vi "BuildRelease_RecompileOpenGDS.vi"() -> ()   [LabVIEW 2020]
uses:
  <vilib>/Utility/config.llb/Read Key (String).vi
  <vilib>/Utility/config.llb/NI_LVConfig.lvlib
panel:
  out "error IO":errorcluster
  out "File":path
  out "Opening":i32
  out "Saving Libraries":i32
  out "Saving Classes":i32
  out "Saving VIs":i32
  out "resulting string":string
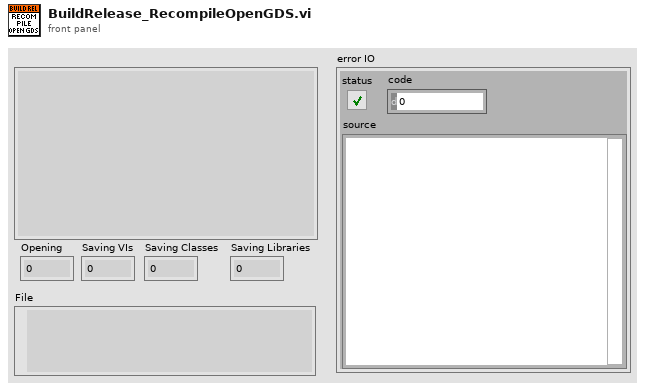
[diagram p1: front panel]
types:
  T1 = cluster{"PID":string, "SpecPath":path, "Files":string[], "BuildPath":path, "InstallerPath":path, "Start":timestamp, "LogFile":path, "AllVIs":refnum<vi>[], "Locked":string[], "Modified":string[], "Bad":string[], "SaveAllError":string[]}
  T2 = enum32{"Bad", "Idle", "Run top level", "Running"}
  T3 = typedef "NI_LVConfig.lvlib/Config Data RefNum.ctl" = refnum<k1>
  T4 = enum32{"invalid lock state", "Not Locked", "Locked (No Password)", "Password-protected"}
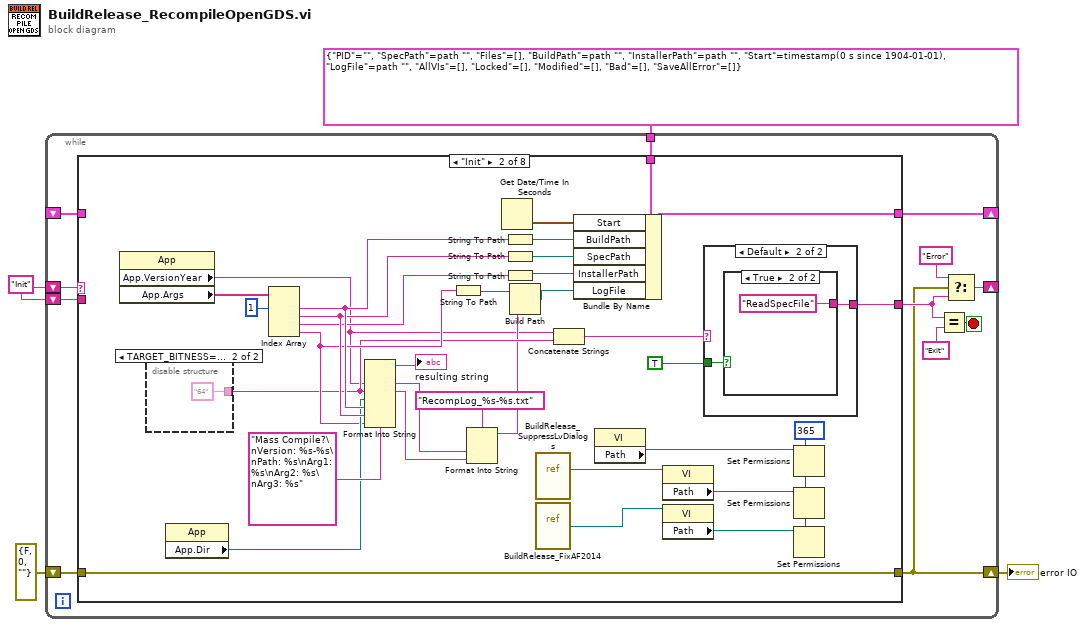
[diagram p0: block diagram]
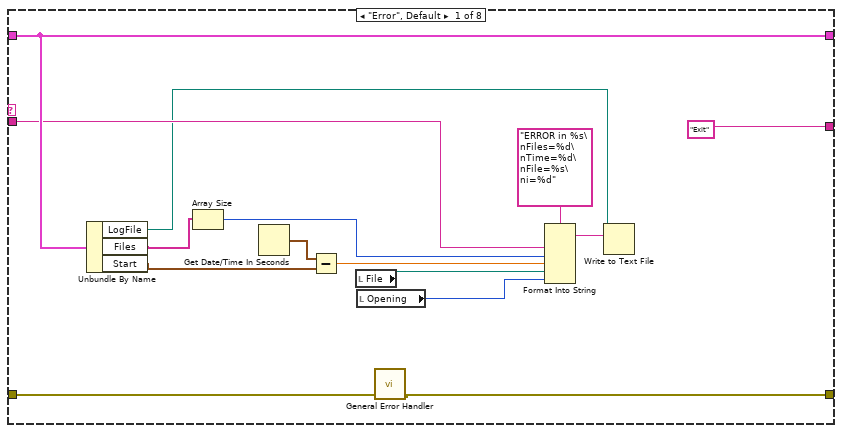
[diagram p2: hidden frame]
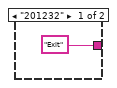
[diagram p3: hidden frame]
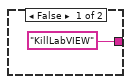
[diagram p4: hidden frame]
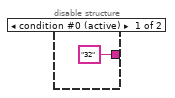
[diagram p5: hidden frame]
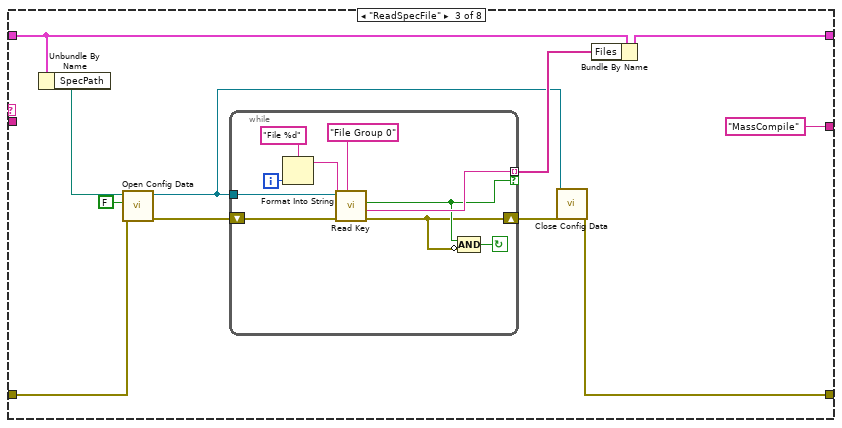
[diagram p6: hidden frame]
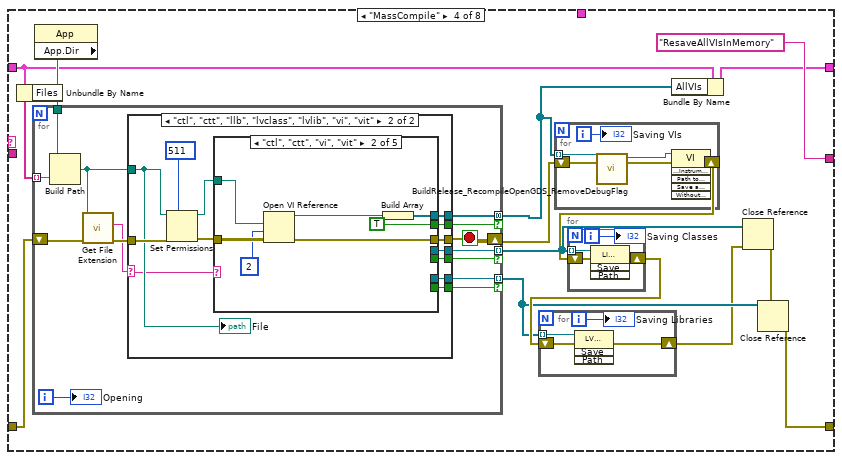
[diagram p7: hidden frame]
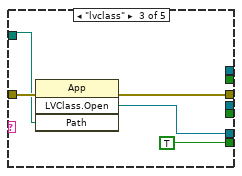
[diagram p10: hidden frame]
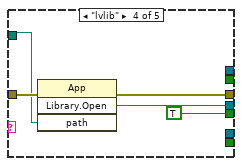
[diagram p11: hidden frame]
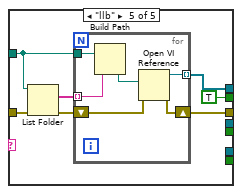
[diagram p12: hidden frame]
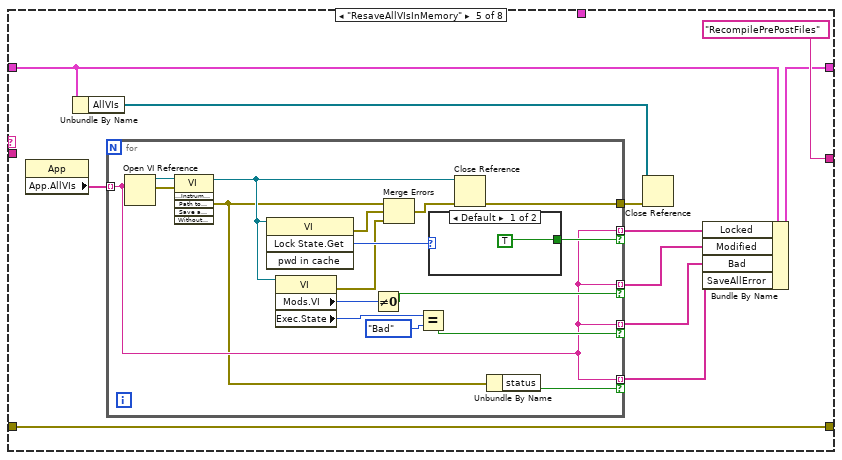
[diagram p13: hidden frame]
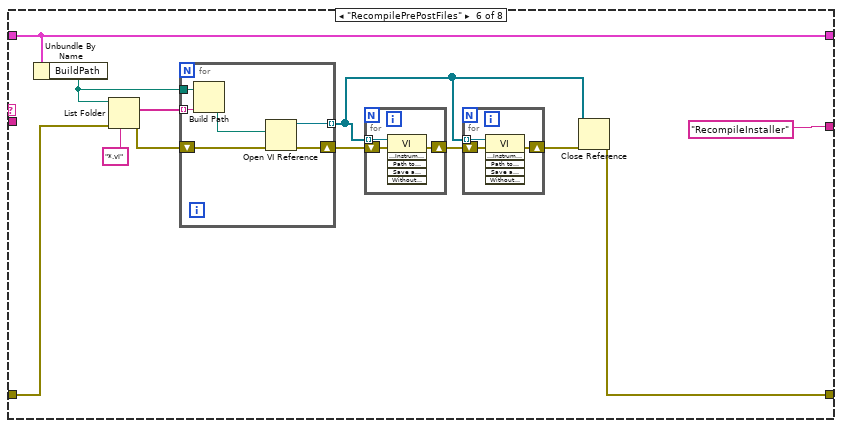
[diagram p15: hidden frame]
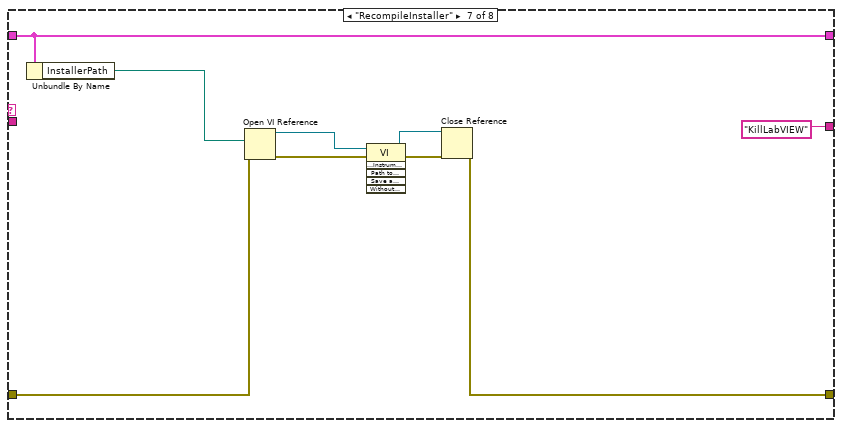
[diagram p16: hidden frame]
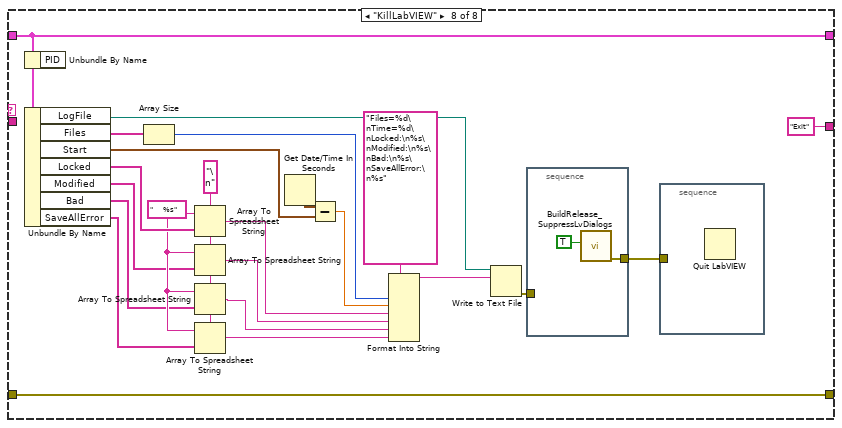
[diagram p17: hidden frame]
diagram:
  w2 = "Init"
  n1 = while {
    shift-right: [w9] -> w1
    shift-left: errorcluster {"status"=FALSE, "code"=0, "source"=""} ("error IO") -> [w16]
    shift-right: [w14] -> _
    shift-left: w2 -> [w15]
    shift-right: [w8] -> _
    shift-left: _ -> [w7]
    tunnel: T1 {"PID"="", "SpecPath"=path "", "Files"=[], "BuildPath"=path "", "InstallerPath"=path "", "Start"=timestamp(0 s since 1904-01-01), "LogFile"=path "", "AllVIs"=[], "Locked"=[], "Modified"=[], "Bad"=[], "SaveAllError"=[]} -> [w6]
    shift-left: w2 -> [w5]
    stop <- w13 stop-if-true
    n2 = case shown="\"Init\"" w15 {
      tunnel: w16 -> [w30 w61 w73 w99 w183 w213 w235 w262]
      tunnel: [w17 w61 w71 w98 w183 w211 w231 w262] -> w9
      tunnel: ["Exit" w62 "MassCompile" "ResaveAllVIsInMemory" "RecompilePrePostFiles" "RecompileInstaller" "KillLabVIEW" "Exit"] -> w10
      tunnel: [w25 w60 w75 w93 w182 w210 w238 w260] -> w8
      tunnel: w7 -> [w25 _ w79 w94 w187 w210 w238 w260]
      tunnel: w6 -> [_ w52 _ _ _ _ _ _]
      tunnel: w5 -> [w21 _ _ _ _ _ _ _]
      frame "Error", Default {
        n3 = Unbundle By Name(w25) -> ("LogFile"=w18:path, "Files"=w23:string[], "Start"=w24:timestamp)
        n4 = Array Size(array=w23) -> (size(s)=w22:i32)
        n5 = Get Date/Time In Seconds() -> (seconds since 1Jan1904=w28:timestamp)
        n6 = Subtract(x=w28, y=w24) -> (x-y=w27:dbl)
        n7 = local read "File"() -> (w20:path)
        n8 = local read "Opening"() -> (w19:i32)
        n9 = call <vilib>:"General Error Handler.vi"("error in (no error)"=w30) -> ("error out"=w17:errorcluster)  [unwired: 10 in, 4 out]
        n10 = Format Into String(format string="ERROR in %s\nFiles=%d\nTime=%d\nFile=%s\ni=%d", w21, w22, w27, w20, w19) -> (resulting string=w26:string)  [unwired: 2 in, 1 out]
        n11 = Write to Text File(file (use dialog)=w18, text=w26) -> ()  [unwired: 2 in, 3 out]
      }
      frame "Init" {
        w33 = i16 365 ("permissions")
        n12 = property class="App"() -> ("App.VersionYear"=w35:string, "App.Args"=w57:string[])  [unwired: 2 in, 2 out]
        n13 = disable-structure shown="TARGET_BITNESS==64" {
          disable-tunnel: ["32" "64"] -> w37
          frame condition #0 (active) {
          }
          frame condition #1 {
          }
        }
        n14 = property class="App"() -> ("App.Dir"=w49:path)  [unwired: 2 in, 2 out]
        n15 = Index Array(array=w57, index #1=1 ("index")) -> (element #1=w55:string, element #2=w54:string, element #3=w43:string, element #4=w41:string)  [unwired: 3 in]
        n16 = Format Into String(format string="Mass Compile?\nVersion: %s-%s\nPath: %s\nArg1: %s\nArg2: %s\nArg3: %s", w35, w37, w49, w55, w54, w41) -> (resulting string=→"resulting string":string)  [unwired: 2 in, 1 out]
        n17 = String To Path(string=w41) -> (path=w40:path)
        n18 = Format Into String(format string="RecompLog_%s-%s.txt", w35, w37) -> (resulting string=w36:string)  [unwired: 2 in, 1 out]
        n19 = Get Date/Time In Seconds() -> (seconds since 1Jan1904=w42:timestamp)
        n20 = String To Path(string=w55) -> (path=w45:path)
        n21 = String To Path(string=w54) -> (path=w53:path)
        n22 = String To Path(string=w43) -> (path=w44:path)
        n23 = Build Path(base path=w40, name or relative path=w36) -> (appended path=w39:path)
        n24 = vi-ref "BuildRelease_SuppressLvDialogs.vi"() -> (w47:refnum<vi>)
        n25 = vi-ref "BuildRelease_FixAF2014.vi"() -> (w32:refnum<vi>)
        n26 = Concatenate Strings(w35, w37) -> (w56:string)
        n27 = Bundle By Name(cluster=w52, "Start"=w42, "BuildPath"=w45, "SpecPath"=w53, "InstallerPath"=w44, "LogFile"=w39) -> (w60:T1)
        n28 = property class="VI"() -> ("Path"=w48:path)  [unwired: 2 in, 2 out]
        n29 = property class="VI"(reference=w47) -> ("Path"=w46:path)  [unwired: 1 in, 2 out]
        n30 = property class="VI"(reference=w32) -> ("Path"=w34:path)  [unwired: 1 in, 2 out]
        n31 = case shown="Default" w56 {
          tunnel: ["Exit" w65] -> w62
          tunnel: TRUE ("T button?") -> [_ w64]
          frame "201232" {
          }
          frame Default {
            n32 = case shown="True" w64 {
              tunnel: ["KillLabVIEW" "ReadSpecFile"] -> w65
              frame False {
              }
              frame True {
              }
            }
          }
        }
        n33 = Set Permissions(7:w33, 11:w48) -> ()  [unwired: 3 in, 2 out]
        n34 = Set Permissions(7:w33, 11:w46) -> ()  [unwired: 3 in, 2 out]
        n35 = Set Permissions(7:w33, 11:w34) -> ()  [unwired: 3 in, 2 out]
      }
      frame "ReadSpecFile" {
        n36 = Unbundle By Name(w79) -> ("SpecPath"=w78:path)
        n37 = call <vilib>:"Open Config Data.vi"("error in (no error)"=w73, "create file if necessary (T)"=FALSE, "configuration file path"=w78) -> ("error out"=w76:errorcluster, "refnum"=w70:T3)  [unwired: 6 in, 1 out]
        n38 = while {
          shift-right: [w82] -> w72
          shift-left: w76 -> [w90]
          tunnel: w70 -> [w89]
          tunnel: [w84] -> w74 mode=indexing if=w83
          i -> [w88]
          stop <- w81 continue-if-true
          n39 = Format Into String(format string="File %d", w88) -> (resulting string=w86:string)  [unwired: 2 in, 1 out]
          n40 = call-poly <vilib>:"Read Key.vi"("section"="File Group 0", "error in (no error)"=w90, "key"=w86, "refnum"=w89) -> ("error out"=w82:errorcluster, "value"=w84:string, "found?"=w83:bool)  [unwired: 4 in, 1 out]
          n41 = Compound Arithmetic op=AND(w83, invert w82) -> (w81:bool)
        }
        n42 = call <vilib>:"Close Config Data.vi"("error in (no error)"=w72, "refnum"=w70) -> ("error out"=w71:errorcluster)  [unwired: 8 in, 1 out]
        n43 = Bundle By Name(cluster=w79, "Files"=w74) -> (w75:T1)
      }
      frame "MassCompile" {
        n44 = Unbundle By Name(w94) -> ("Files"=w95:string[])
        n45 = property class="App"() -> ("App.Dir"=w97:path)  [unwired: 2 in, 2 out]
        n46 = for {
          tunnel: w95 -> [w126] mode=indexing
          tunnel: [w132] -> w92 mode=concatenating if=w131
          shift-right: [w123] -> w96
          shift-left: w99 -> [w122]
          tunnel: [w130] -> w102 mode=indexing if=w129
          tunnel: [w128] -> w101 mode=indexing if=w127
          tunnel: w97 -> [w125]
          i -> [w124]
          stop <- w123 stop-if-true
          n47 = Build Path(base path=w125, name or relative path=w126) -> (appended path=w120:path)
          n48 = call <vilib>:"Get File Extension.vi"("error in (no error)"=w122, "file"=w120) -> ("error out"=w121:errorcluster, "lowercase file extension"=w119:string)  [unwired: 5 in, 3 out]
          n49 = case shown="\"ctl\", \"ctt\", \"llb\", \"lvclass\", \"lvlib\", \"vi\", \"vit\"" w119 {
            selector: w119 -> [_ w134]
            tunnel: [_ w146] -> w132
            tunnel: [_ w145] -> w131
            tunnel: [_ w144] -> w130
            tunnel: [_ w143] -> w129
            tunnel: [_ w142] -> w128
            tunnel: [_ w141] -> w127
            tunnel: [w133 w139] -> w123
            tunnel: w121 -> [w133 w136]
            tunnel: w120 -> [_ w135]
            frame Default {
            }
            frame "ctl", "ctt", "llb", "lvclass", "lvlib", "vi", "vit" {
              n50 = Set Permissions(7:i16 511 ("permissions"), 8:w136, 11:w135) -> (0:w140:errorcluster, 3:w138:path)  [unwired: 2 in]
              n51 = case shown="\"ctl\", \"ctt\", \"vi\", \"vit\"" w134 {
                tunnel: w140 -> [w147 w154 w159 w164 w166]
                tunnel: w138 -> [_ w153 w158 w163 w165]
                tunnel: [_ w149 _ _ w171] -> w146
                tunnel: [_ TRUE _ _ TRUE] -> w145
                tunnel: [w147 w150 w157 w160 w169] -> w139
                tunnel: [_ _ _ w162 _] -> w144
                tunnel: [_ _ _ TRUE _] -> w143
                tunnel: [_ _ w156 _ _] -> w142
                tunnel: [_ _ TRUE _ _] -> w141
                frame Default {
                }
                frame "ctl", "ctt", "vi", "vit" {
                  n52 = Open VI Reference(vi path=w153, options=2, error in (no error)=w154) -> (vi reference=w152:refnum<vi>, error out=w150:errorcluster)  [unwired: 3 in]
                  n53 = Build Array(w152) -> (w149:refnum<vi>[])
                }
                frame "lvclass" {
                  n54 = invoke class="App" method="LVClass.Open"(error in=w159, "Path"=w158) -> (error out=w157:errorcluster, "LVClass.Open"=w156:refnum<vi>)  [unwired: 2 in, 2 out]
                }
                frame "lvlib" {
                  n55 = invoke class="App" method="Library.Open"(error in=w164, "path"=w163) -> (error out=w160:errorcluster, "Open Library"=w162:refnum<vi>)  [unwired: 2 in, 2 out]
                }
                frame "llb" {
                  n56 = List Folder(path=w165, error in=w166) -> (filenames=w167:string[], error out=w168:errorcluster)  [unwired: 1 in, 3 out]
                  n57 = for {
                    tunnel: w167 -> [w172] mode=indexing
                    tunnel: w165 -> [w177]
                    shift-right: [w174] -> w169
                    shift-left: w168 -> [w175]
                    tunnel: [w173] -> w171 mode=indexing
                    n58 = Build Path(base path=w177, name or relative path=w172) -> (appended path=w176:path)
                    n59 = Open VI Reference(vi path=w176, error in (no error)=w175) -> (vi reference=w173:refnum<vi>, error out=w174:errorcluster)  [unwired: 4 in]
                  }
                }
              }
              "File" <- w135
            }
          }
          "Opening" <- w124
        }
        n60 = for {
          tunnel: w92 -> [w118] mode=indexing
          shift-right: [w116] -> w104
          shift-left: w96 -> [w117]
          i -> [w115]
          n61 = call "BuildRelease_RecompileOpenGDS_RemoveDebugFlag.vi"("VI in"=w118) -> ("VI out"=w114:refnum<vi>)  [unwired: 10 in]
          n62 = invoke class="VI" method="Save.Instrument"(reference=w114, error in=w117) -> (error out=w116:errorcluster)  [unwired: 4 in, 5 out]
          "Saving VIs" <- w115
        }
        n63 = for {
          tunnel: w102 -> [w113] mode=indexing
          shift-right: [w111] -> w103
          shift-left: w104 -> [w112]
          i -> [w110]
          n64 = invoke class="Library" method="Save"(reference=w113, error in=w112) -> (error out=w111:errorcluster)  [unwired: 2 in, 3 out]
          "Saving Classes" <- w110
        }
        n65 = for {
          tunnel: w101 -> [w109] mode=indexing
          shift-right: [w107] -> w91
          shift-left: w103 -> [w108]
          i -> [w106]
          n66 = invoke class="LVClassLibrary" method="Save"(reference=w109, error in=w108) -> (error out=w107:errorcluster)  [unwired: 2 in, 3 out]
          "Saving Libraries" <- w106
        }
        n67 = Bundle By Name(cluster=w94, "AllVIs"=w92) -> (w93:T1)
        n68 = Close Reference(reference=w102, error in (no error)=w91) -> (error out=w100:errorcluster)
        n69 = Close Reference(reference=w101, error in (no error)=w100) -> (error out=w98:errorcluster)
      }
      frame "ResaveAllVIsInMemory" {
        n70 = property class="App"() -> ("App.AllVIs"=w186:string[])  [unwired: 2 in, 2 out]
        n71 = Unbundle By Name(w187) -> ("AllVIs"=w184:refnum<vi>[])
        n72 = for {
          tunnel: w186 -> [w194] mode=indexing
          tunnel: [w203] -> w185
          tunnel: [w194] -> w181 mode=indexing if=w197
          tunnel: [w194] -> w180 mode=indexing if=w196
          tunnel: [w194] -> w179 mode=indexing if=w195
          tunnel: [w194] -> w178 mode=indexing if=w192
          n73 = Open VI Reference(vi path=w194) -> (vi reference=w205:refnum<vi>, error out=w204:errorcluster)  [unwired: 5 in]
          n74 = invoke class="VI" method="Save.Instrument"(reference=w205, error in=w204) -> (reference out=w198:refnum<vi>, error out=w193:errorcluster)  [unwired: 4 in, 4 out]
          n75 = invoke class="VI" method="Lock State.Get"(reference=w198) -> (error out=w190:errorcluster, "Get Lock State"=w199:T4)  [unwired: 3 in, 2 out]
          n76 = property class="VI"(reference=w198) -> (error out=w189:errorcluster, "Mods.VI"=w202:u64, "Exec.State"=w201:T2)  [unwired: 1 in, 1 out]
          n77 = Not Equal To 0?(x=w202) -> (x != 0?=w196:bool)
          n78 = Merge Errors(w193, w190, w189) -> (w191:errorcluster)
          n79 = Equal?(x=w201, y=T2."Bad") -> (x = y?=w195:bool)
          n80 = case shown="Default" w199 {
            tunnel: [TRUE _] -> w197
            frame Default {
            }
            frame "invalid lock state", "Not Locked" {
            }
          }
          n81 = Close Reference(reference=w198, error in (no error)=w191) -> (error out=w203:errorcluster)
          n82 = Unbundle By Name(w193) -> ("status"=w192:bool)
        }
        n83 = Close Reference(reference=w184, error in (no error)=w185) -> ()  [unwired: 1 out]
        n84 = Bundle By Name(cluster=w187, "Locked"=w181, "Modified"=w180, "Bad"=w179, "SaveAllError"=w178) -> (w182:T1)
      }
      frame "RecompilePrePostFiles" {
        n85 = Unbundle By Name(w210) -> ("BuildPath"=w216:path)
        n86 = List Folder(path=w216, pattern="*.vi", error in=w213) -> (filenames=w215:string[], error out=w214:errorcluster)  [unwired: 1 in, 2 out]
        n87 = for {
          tunnel: w216 -> [w230]
          tunnel: w215 -> [w229] mode=indexing
          tunnel: [w226] -> w207 mode=indexing
          shift-right: [w225] -> w212
          shift-left: w214 -> [w227]
          n88 = Build Path(base path=w230, name or relative path=w229) -> (appended path=w228:path)
          n89 = Open VI Reference(vi path=w228, error in (no error)=w227) -> (vi reference=w226:refnum<vi>, error out=w225:errorcluster)  [unwired: 4 in]
        }
        n90 = for {
          tunnel: w207 -> [w224] mode=indexing
          shift-right: [w222] -> w209
          shift-left: w212 -> [w223]
          n91 = invoke class="VI" method="Save.Instrument"(reference=w224, error in=w223) -> (error out=w222:errorcluster)  [unwired: 4 in, 5 out]
        }
        n92 = for {
          tunnel: w207 -> [w221] mode=indexing
          shift-right: [w219] -> w208
          shift-left: w209 -> [w220]
          n93 = invoke class="VI" method="Save.Instrument"(reference=w221, error in=w220) -> (error out=w219:errorcluster)  [unwired: 4 in, 5 out]
        }
        n94 = Close Reference(reference=w207, error in (no error)=w208) -> (error out=w211:errorcluster)
      }
      frame "RecompileInstaller" {
        n95 = Unbundle By Name(w238) -> ("InstallerPath"=w236:path)
        n96 = Open VI Reference(vi path=w236, error in (no error)=w235) -> (vi reference=w232:refnum<vi>, error out=w234:errorcluster)  [unwired: 4 in]
        n97 = invoke class="VI" method="Save.Instrument"(reference=w232, error in=w234) -> (reference out=w233:refnum<vi>, error out=w237:errorcluster)  [unwired: 4 in, 4 out]
        n98 = Close Reference(reference=w233, error in (no error)=w237) -> (error out=w231:errorcluster)
      }
      frame "KillLabVIEW" {
        w246 = "     %s" ("delimiter (Tab)")
        w247 = "\n" ("delimiter (Tab)")
        n99 = Unbundle By Name(w260) -> ()  [unwired: 1 out]
        n100 = Unbundle By Name(w260) -> ("LogFile"=w251:path, "Files"=w253:string[], "Start"=w255:timestamp, "Locked"=w249:string[], "Modified"=w245:string[], "Bad"=w244:string[], "SaveAllError"=w243:string[])
        n101 = Array Size(array=w253) -> (size(s)=w252:i32)
        n102 = Array To Spreadsheet String(delimiter (Tab)=w247, array=w249, 3:w246) -> (spreadsheet string=w248:string)
        n103 = Array To Spreadsheet String(delimiter (Tab)=w247, array=w245, 3:w246) -> (spreadsheet string=w242:string)
        n104 = Array To Spreadsheet String(delimiter (Tab)=w247, array=w244, 3:w246) -> (spreadsheet string=w241:string)
        n105 = Array To Spreadsheet String(delimiter (Tab)=w247, array=w243, 3:w246) -> (spreadsheet string=w240:string)
        n106 = Get Date/Time In Seconds() -> (seconds since 1Jan1904=w256:timestamp)
        n107 = Subtract(x=w256, y=w255) -> (x-y=w254:dbl)
        n108 = Format Into String(format string="Files=%d\nTime=%d\nLocked:\n%s\nModified:\n%s\nBad:\n%s\nSaveAllError:\n%s", w252, w254, w248, w242, w241, w240) -> (resulting string=w250:string)  [unwired: 2 in, 1 out]
        n109 = Write to Text File(file (use dialog)=w251, text=w250) -> (error out=w258:errorcluster)  [unwired: 2 in, 2 out]
        n110 = stacked-sequence {
          tunnel: [w263] -> w259
          tunnel: w258 -> [_]
          frame #0 {
            n111 = call "BuildRelease_SuppressLvDialogs.vi"("Suppress Dialogs? (F)"=TRUE) -> ("error out"=w263:errorcluster)  [unwired: 10 in]
          }
        }
        n112 = stacked-sequence {
          tunnel: w259 -> [_]
          frame #0 {
            n113 = Quit LabVIEW() -> ()  [unwired: 1 in]
          }
        }
      }
    }
    n114 = Equal?(x=w10, y="Exit") -> (x = y?=w13:bool)
    n115 = Select(t="Error", s=w9, f=w10) -> (s? t:f=w14:string)
  }
  "error IO" <- w1
